vi "ArbRampGenerator.vi"() -> ()   [LabVIEW 2010]
panel:
  out "Waveform Graph":dbl[](graph)
  out "Samples/Cycle":dbl
  out "Sample Rate":dbl
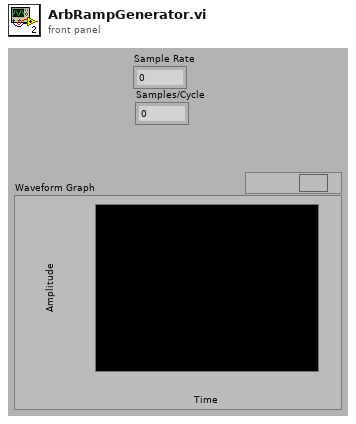
[diagram p1: front panel]
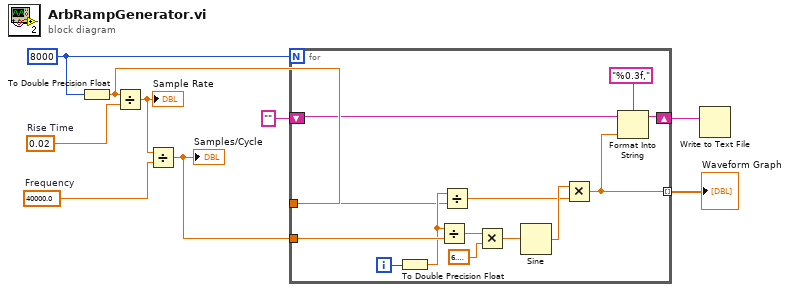
[diagram p0: block diagram]
diagram:
  w6 = 40000.0  # Frequency
  w8 = 0.02  # Rise Time
  w9 = 8000
  n1 = To Double Precision Float(number=w9) -> (double precision float=w3:dbl)
  n2 = Divide(x=w3, y=w8) -> (x/y=w7:dbl)
  "Sample Rate" <- w7
  n3 = Divide(x=w7, y=w6) -> (x/y=w5:dbl)
  "Samples/Cycle" <- w5
  n4 = for {
    N: w9 -> [_]
    tunnel: w5 -> [w21]
    tunnel: [w10] -> w4 mode=indexing
    tunnel: w3 -> [w15]
    shift-right: [w11] -> w1
    shift-left: "" -> [w13]
    i -> [w22]
    n5 = To Double Precision Float(number=w22) -> (double precision float=w16:dbl)
    n6 = Divide(x=w16, y=w21) -> (x/y=w19:dbl)
    n7 = Divide(x=w16, y=w15) -> (x/y=w14:dbl)
    n8 = Multiply(x=w19, y=6.283185307179586) -> (x*y=w18:dbl)
    n9 = Sine(x=w18) -> (sin(x)=w17:dbl)
    n10 = Multiply(x=w17, y=w14) -> (x*y=w10:dbl)
    n11 = Format Into String(format string="%0.3f,", initial string=w13, w10) -> (resulting string=w11:string)  [unwired: 1 in, 1 out]
  }
  "Waveform Graph" <- w4
  n12 = Write to Text File(text=w1) -> ()  [unwired: 3 in, 3 out]
